vi "HandleSuffix.vi"(8 "error in (no error)":errorcluster, 11 "S4GUI in":refnum<class "S4GUI.lvclass">) -> (0 "error out":errorcluster, 3 "S4GUI out":refnum<class "S4GUI.lvclass">)   [LabVIEW 2018, in "S4GUI.lvclass"]
uses:
  S4GUI.lvclass
  S4GUI.lvclass/S4GUI.ctl
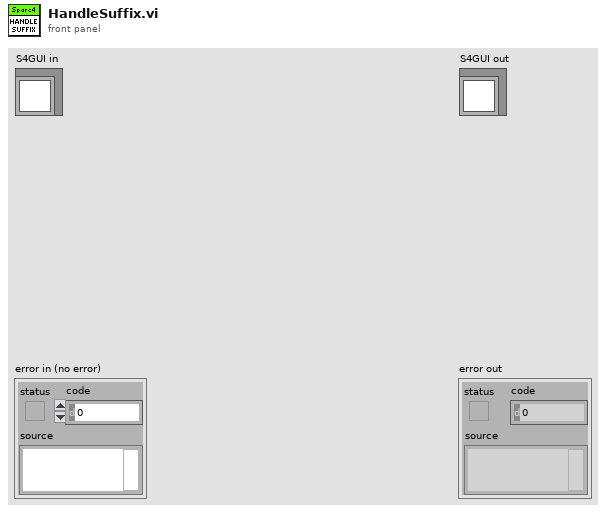
[diagram p1: front panel]
types:
  T1 = enum32{"OBJECT", "DFLAT", "SFLAT", "DARK", "ZERO", "FOCUS"}
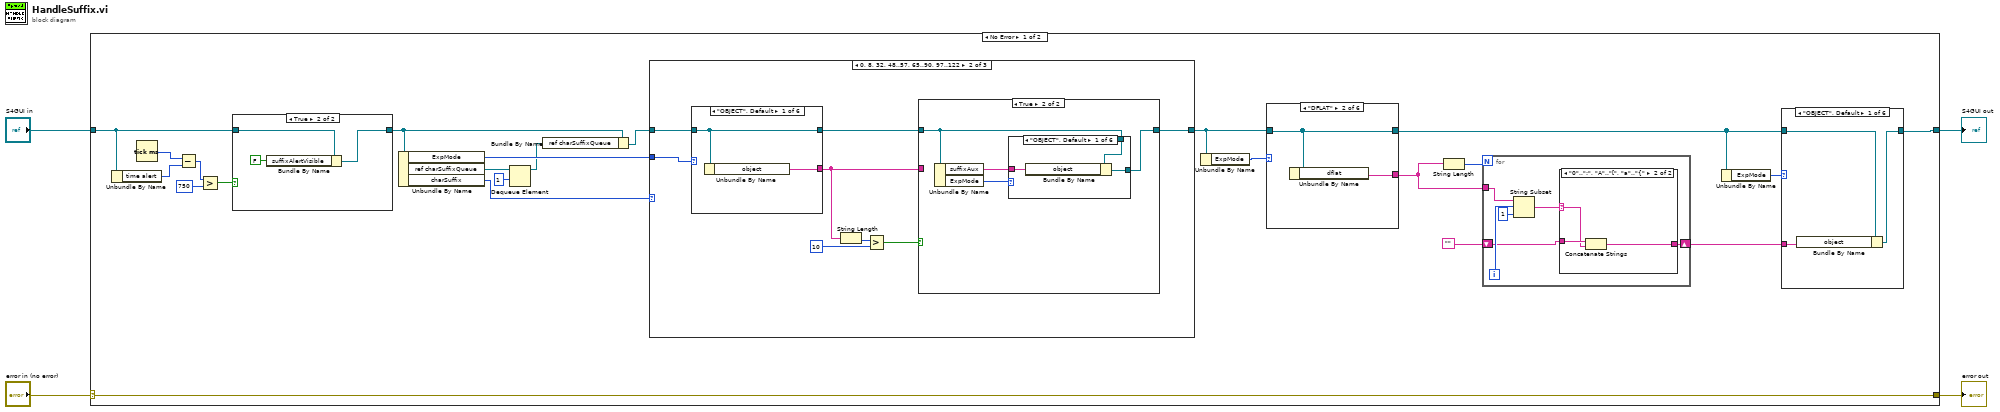
[diagram p0: block diagram]
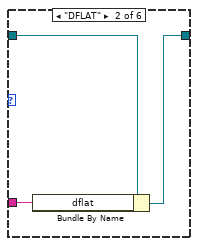
[diagram p2: hidden frame]
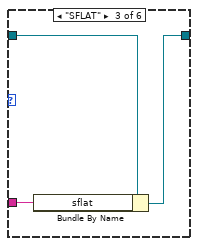
[diagram p3: hidden frame]
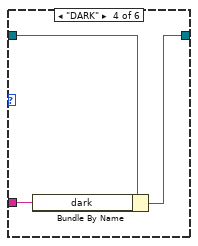
[diagram p4: hidden frame]
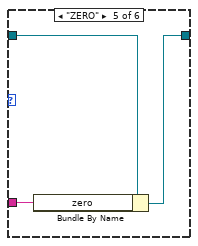
[diagram p5: hidden frame]
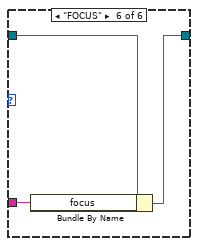
[diagram p6: hidden frame]
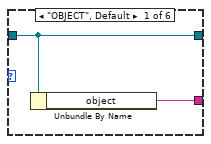
[diagram p8: hidden frame]
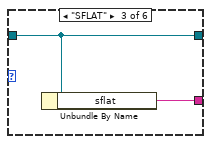
[diagram p9: hidden frame]
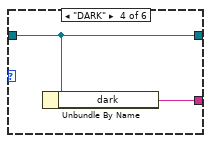
[diagram p10: hidden frame]
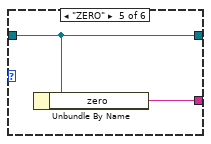
[diagram p11: hidden frame]
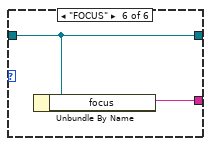
[diagram p12: hidden frame]
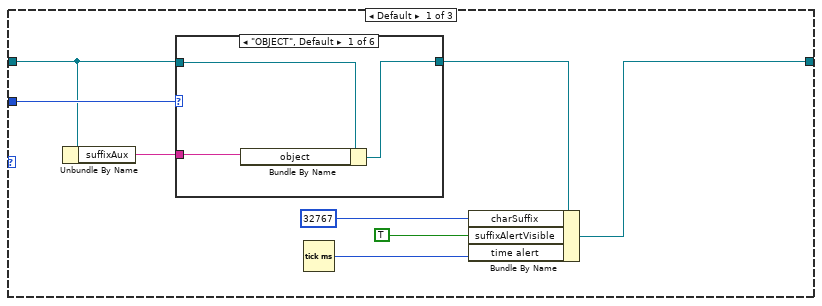
[diagram p13: hidden frame]
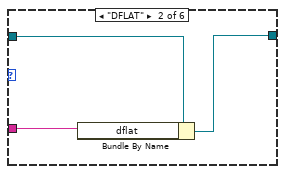
[diagram p14: hidden frame]
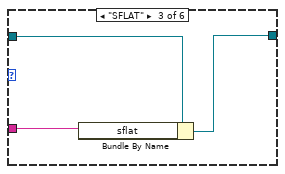
[diagram p15: hidden frame]
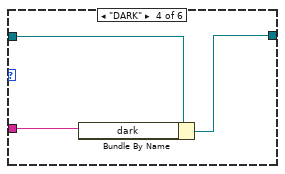
[diagram p16: hidden frame]
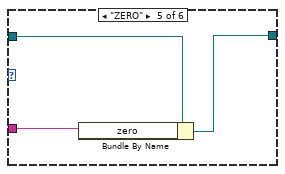
[diagram p17: hidden frame]
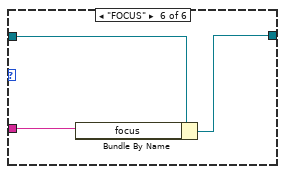
[diagram p18: hidden frame]
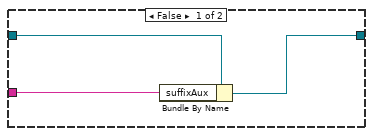
[diagram p19: hidden frame]
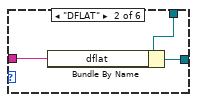
[diagram p20: hidden frame]
diagram:
  n1 = case shown="No Error" "error in (no error)" {
    selector: "error in (no error)" -> [w27 w145]
    tunnel: [w27 w145] -> w3
    tunnel: [w6 w144] -> w1
    tunnel: "S4GUI in" -> [w22 w144]
    frame No Error {
      n2 = Unbundle By Name(w22) -> ("time alert"=w24:u32)
      n3 = Tick Count (ms)() -> (millisecond timer value=w25:u32)
      n4 = Subtract(x=w25, y=w24) -> (x-y=w26:u32)
      n5 = Greater?(x=w26, y=u32 750) -> (0:w21:bool)
      n6 = case shown="True" w21 {
        tunnel: w22 -> [w140 w143]
        tunnel: [w140 w142] -> w18
        frame False {
        }
        frame True {
          n7 = Bundle By Name(cluster=w143, "suffixAlertVisible"=FALSE) -> (w142:refnum<class "S4GUI.lvclass">)
        }
      }
      n8 = Unbundle By Name(w18) -> ("ExpMode"=w20:T1, "ref charSuffixQueue"=w19:refnum<queue>, "charSuffix"=w14:i16)
      n9 = Dequeue Element(queue=w19, timeout in ms (-1)=1) -> (queue out=w16:refnum<queue>)  [unwired: 1 in, 3 out]
      n10 = Bundle By Name(cluster=w18, "ref charSuffixQueue"=w16) -> (w17:refnum<class "S4GUI.lvclass">)
      n11 = case shown="0, 8, 32, 48..57, 65..90, 97..122" w14 {
        tunnel: w17 -> [w74 w101 w139]
        tunnel: w20 -> [w75 w100 _]
        tunnel: [w68 w95 w139] -> w12
        frame Default {
          n12 = Unbundle By Name(w74) -> ("suffixAux"=w73:string)
          n13 = case shown="\"OBJECT\", Default" w75 {
            tunnel: w74 -> [w78 w81 w84 w87 w90 w93]
            tunnel: [w77 w80 w83 w86 w89 w92] -> w72
            tunnel: w73 -> [w76 w79 w82 w85 w88 w91]
            frame "OBJECT", Default {
              n14 = Bundle By Name(cluster=w78, "object"=w76) -> (w77:refnum<class "S4GUI.lvclass">)
            }
            frame "DFLAT" {
              n15 = Bundle By Name(cluster=w81, "dflat"=w79) -> (w80:refnum<class "S4GUI.lvclass">)
            }
            frame "SFLAT" {
              n16 = Bundle By Name(cluster=w84, "sflat"=w82) -> (w83:refnum<class "S4GUI.lvclass">)
            }
            frame "DARK" {
              n17 = Bundle By Name(cluster=w87, "dark"=w85) -> (w86:refnum<class "S4GUI.lvclass">)
            }
            frame "ZERO" {
              n18 = Bundle By Name(cluster=w90, "zero"=w88) -> (w89:refnum<class "S4GUI.lvclass">)
            }
            frame "FOCUS" {
              n19 = Bundle By Name(cluster=w93, "focus"=w91) -> (w92:refnum<class "S4GUI.lvclass">)
            }
          }
          n20 = Tick Count (ms)() -> (millisecond timer value=w69:u32)
          n21 = Bundle By Name(cluster=w72, "charSuffix"=i16 32767, "suffixAlertVisible"=TRUE, "time alert"=w69) -> (w68:refnum<class "S4GUI.lvclass">)
        }
        frame 0, 8, 32, 48..57, 65..90, 97..122 {
          n22 = case shown="\"OBJECT\", Default" w100 {
            tunnel: w101 -> [w128 w130 w132 w134 w136 w138]
            tunnel: [w128 w130 w132 w134 w136 w138] -> w96
            tunnel: [w127 w129 w131 w133 w135 w137] -> w94
            frame "OBJECT", Default {
              n23 = Unbundle By Name(w128) -> ("object"=w127:string)
            }
            frame "DFLAT" {
              n24 = Unbundle By Name(w130) -> ("dflat"=w129:string)
            }
            frame "SFLAT" {
              n25 = Unbundle By Name(w132) -> ("sflat"=w131:string)
            }
            frame "DARK" {
              n26 = Unbundle By Name(w134) -> ("dark"=w133:string)
            }
            frame "ZERO" {
              n27 = Unbundle By Name(w136) -> ("zero"=w135:string)
            }
            frame "FOCUS" {
              n28 = Unbundle By Name(w138) -> ("focus"=w137:string)
            }
          }
          n29 = String Length(string=w94) -> (length=w99:i32)
          n30 = Greater?(x=w99, y=10) -> (0:w97:bool)
          n31 = case shown="True" w97 {
            tunnel: w96 -> [w104 w108]
            tunnel: [w103 w107] -> w95
            tunnel: w94 -> [w102 _]
            frame False {
              n32 = Bundle By Name(cluster=w104, "suffixAux"=w102) -> (w103:refnum<class "S4GUI.lvclass">)
            }
            frame True {
              n33 = Unbundle By Name(w108) -> ("suffixAux"=w105:string, "ExpMode"=w106:T1)
              n34 = case shown="\"OBJECT\", Default" w106 {
                tunnel: w108 -> [w111 w114 w117 w120 w123 w125]
                tunnel: [w110 w113 w116 w119 w122 w124] -> w107
                tunnel: w105 -> [w109 w112 w115 w118 w121 w126]
                frame "OBJECT", Default {
                  n35 = Bundle By Name(cluster=w111, "object"=w109) -> (w110:refnum<class "S4GUI.lvclass">)
                }
                frame "DFLAT" {
                  n36 = Bundle By Name(cluster=w114, "dflat"=w112) -> (w113:refnum<class "S4GUI.lvclass">)
                }
                frame "SFLAT" {
                  n37 = Bundle By Name(cluster=w117, "sflat"=w115) -> (w116:refnum<class "S4GUI.lvclass">)
                }
                frame "DARK" {
                  n38 = Bundle By Name(cluster=w120, "dark"=w118) -> (w119:refnum<class "S4GUI.lvclass">)
                }
                frame "ZERO" {
                  n39 = Bundle By Name(cluster=w123, "zero"=w121) -> (w122:refnum<class "S4GUI.lvclass">)
                }
                frame "FOCUS" {
                  n40 = Bundle By Name(cluster=w125, "focus"=w126) -> (w124:refnum<class "S4GUI.lvclass">)
                }
              }
            }
          }
        }
        frame 32767 {
        }
      }
      n41 = Unbundle By Name(w12) -> ("ExpMode"=w13:T1)
      n42 = case shown="\"DFLAT\"" w13 {
        tunnel: w12 -> [w57 w59 w61 w63 w65 w67]
        tunnel: [w56 w58 w60 w62 w64 w66] -> w10
        tunnel: [w57 w59 w61 w63 w65 w67] -> w7
        frame "OBJECT", Default {
          n43 = Unbundle By Name(w57) -> ("object"=w56:string)
        }
        frame "DFLAT" {
          n44 = Unbundle By Name(w59) -> ("dflat"=w58:string)
        }
        frame "SFLAT" {
          n45 = Unbundle By Name(w61) -> ("sflat"=w60:string)
        }
        frame "DARK" {
          n46 = Unbundle By Name(w63) -> ("dark"=w62:string)
        }
        frame "ZERO" {
          n47 = Unbundle By Name(w65) -> ("zero"=w64:string)
        }
        frame "FOCUS" {
          n48 = Unbundle By Name(w67) -> ("focus"=w66:string)
        }
      }
      n49 = String Length(string=w10) -> (length=w11:i32)
      n50 = for {
        N: w11 -> [_]
        tunnel: w10 -> [w51]
        shift-right: [w46] -> w5
        shift-left: "" -> [w48]
        i -> [w50]
        n51 = String Subset(string=w51, offset (0)=w50, length (rest)=1 ("length (rest)")) -> (substring=w47:string)
        n52 = case shown="\"0\"..\":\", \"A\"..\"[\", \"a\"..\"{\"" w47 {
          selector: w47 -> [_ w54]
          tunnel: w48 -> [w52 w55]
          tunnel: [w52 w53] -> w46
          frame Default {
          }
          frame "0"..":", "A".."[", "a".."{" {
            n53 = Concatenate Strings(w55, w54) -> (w53:string)
          }
        }
      }
      n54 = Unbundle By Name(w7) -> ("ExpMode"=w8:T1)
      n55 = case shown="\"OBJECT\", Default" w8 {
        tunnel: w7 -> [w30 w33 w36 w39 w42 w45]
        tunnel: [w29 w32 w35 w38 w41 w44] -> w6
        tunnel: w5 -> [w28 w31 w34 w37 w40 w43]
        frame "OBJECT", Default {
          n56 = Bundle By Name(cluster=w30, "object"=w28) -> (w29:refnum<class "S4GUI.lvclass">)
        }
        frame "DFLAT" {
          n57 = Bundle By Name(cluster=w33, "dflat"=w31) -> (w32:refnum<class "S4GUI.lvclass">)
        }
        frame "SFLAT" {
          n58 = Bundle By Name(cluster=w36, "sflat"=w34) -> (w35:refnum<class "S4GUI.lvclass">)
        }
        frame "DARK" {
          n59 = Bundle By Name(cluster=w39, "dark"=w37) -> (w38:refnum<class "S4GUI.lvclass">)
        }
        frame "ZERO" {
          n60 = Bundle By Name(cluster=w42, "zero"=w40) -> (w41:refnum<class "S4GUI.lvclass">)
        }
        frame "FOCUS" {
          n61 = Bundle By Name(cluster=w45, "focus"=w43) -> (w44:refnum<class "S4GUI.lvclass">)
        }
      }
    }
    frame Error {
    }
  }
  "error out" <- w3
  "S4GUI out" <- w1
